vi "Chronometer.vi"(1 "start":bool, 2 "reset":bool) -> (0 "Time":dbl)   [LabVIEW 2014]
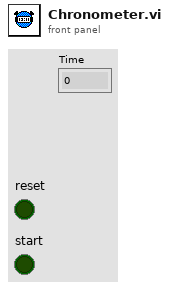
[diagram p1: front panel]
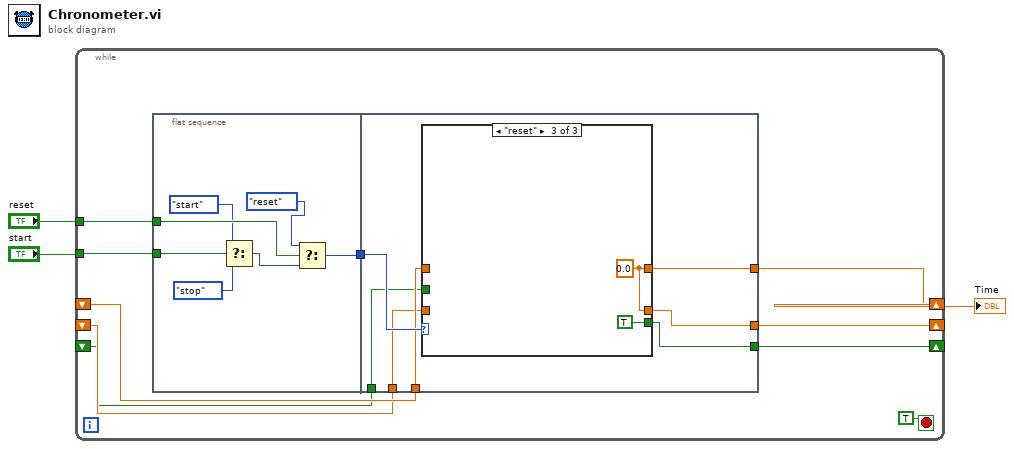
[diagram p0: block diagram]
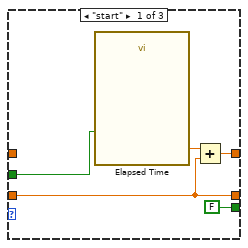
[diagram p2: hidden frame]
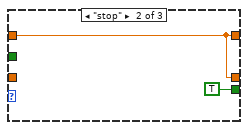
[diagram p3: hidden frame]
diagram:
  n1 = while {
    shift-right: [w10] -> w3
    shift-left: _ -> [w6]
    shift-right: [w9] -> _
    shift-left: _ -> [w5]
    shift-right: [w8] -> _
    shift-left: _ -> [w4]
    tunnel: "start" -> [w12]
    tunnel: "reset" -> [w11]
    stop <- TRUE stop-if-true
    n2 = flat-sequence {
      tunnel: w12 -> [w19]
      tunnel: w11 -> [w18]
      tunnel: [w14] -> w7
      tunnel: [w27] -> w10
      tunnel: [w26] -> w9
      tunnel: [w25] -> w8
      tunnel: w7 -> [w24]
      tunnel: w6 -> [w23]
      tunnel: w5 -> [w22]
      tunnel: w4 -> [w21]
      frame #0 {
        n3 = Select(t=enum16{"start", "stop", "reset"}."start" ("action"), s=w19, f=enum16{"start", "stop", "reset"}."stop" ("action")) -> (s? t:f=w17:enum16{"start", "stop", "reset"})
        n4 = Select(t=enum16{"start", "stop", "reset"}."reset" ("action"), s=w18, f=w17) -> (s? t:f=w14:enum16{"start", "stop", "reset"})
      }
      frame #1 {
        n5 = case shown="\"reset\"" w24 {
          tunnel: [w30 w33 w35] -> w27
          tunnel: w23 -> [_ w33 _]
          tunnel: w21 -> [w31 _ _]
          tunnel: [FALSE TRUE TRUE] -> w25
          tunnel: w22 -> [w29 _ _]
          tunnel: [w29 w33 w35] -> w26
          frame "start" {
            n6 = call "Elapsed Time"("Reset"=w31) -> ("Elapsed Time (s)"=w32:dbl)  [unwired: 11 in, 7 out]
            n7 = Add(x=w32, y=w29) -> (x+y=w30:dbl)
          }
          frame "stop" {
          }
          frame "reset" {
            w35 = 0.0 ("Elapsed Time (s)")
          }
        }
      }
    }
  }
  "Time" <- w3
